vi "Get Relevant Table of Pressures.vi"(3 "Length of List for 1 Pressure":i32, 4 "Psych Table":dbl[][](array[numeric])=array4950x10[49500 elements], 5 "Air Pressure [psia]":dbl) -> (0 "Pressure Index":dbl, 1 "Lower Pressure Psych Table":dbl[][](array[numeric]), 2 "Higher Pressure Psych Table":dbl[][](array[numeric]))   [LabVIEW 2020]
panel:
  # "THIS IS THE NUMBER OF ROWS CONTAINED\nIN ALL OF THE ENTRIES FOR EACH PRESSURE\n(ONLY WORKS IF EACH LENGTH IS THE SAME \nIN THE LIST)"
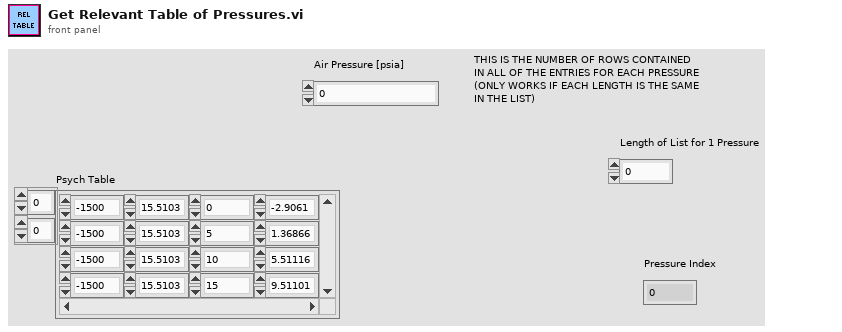
[diagram p1: front panel]
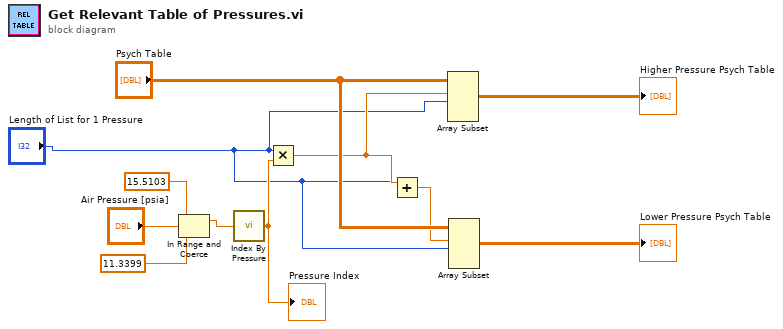
[diagram p0: block diagram]
diagram:
  n1 = In Range and Coerce(upper limit=15.5103, x="Air Pressure [psia]", lower limit=11.3399) -> (coerced(x)=w4:dbl)  [unwired: 1 out]
  n2 = call "Index By Pressure.vi"("Air Pressure [psia]"=w4) -> ("Pressure Index"=w10:dbl)
  "Pressure Index" <- w10
  n3 = Multiply(x="Length of List for 1 Pressure", y=w10) -> (x*y=w8:dbl)
  n4 = Add(x=w8, y="Length of List for 1 Pressure") -> (x+y=w7:dbl)
  n5 = Array Subset(array="Psych Table", index (row)=w8, length (row)="Length of List for 1 Pressure") -> (→"Higher Pressure Psych Table":dbl[][])  [unwired: 2 in]
  n6 = Array Subset(array="Psych Table", index (row)=w7, length (row)="Length of List for 1 Pressure") -> (→"Lower Pressure Psych Table":dbl[][])  [unwired: 2 in]
